vi "example_dynamically_invoking - slave.vi"() -> ()   [LabVIEW 2012]
doc: "This is the Slave VI that is called upon by the controlling Master (example_dynamically_invoking - master.vi). This VI is responsible for handling the communications with the attached hardware while the controlling Master simply issues the appropriate action calls to this one.\n\nProduced By:\n\nChristopher Lemieux\nKod Integrations, LLC\n4835 Marianne Drive\nMount Airy, MD 21771\nhttp://www.kodintegrations.com\nemail: clemieux@kodintegrations.com\nphone: (240) 687-1288"
uses:
  controls/example_dynamically_invoking - slave_actions.ctl
  main_functions/commands.ctl
panel:
  in  "slave_action":T1=enum."initialize"
  out "error out":errorcluster
  in  "error in (no error)":errorcluster
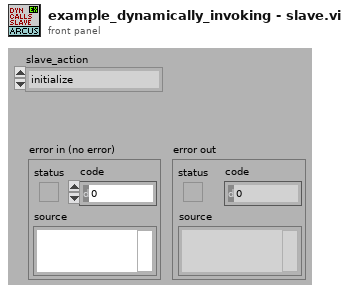
[diagram p1: front panel]
types:
  T1 = typedef "example_dynamically_invoking - slave_actions.ctl" = enum16{"exit", "initialize", "jogConstNeg", "jogConstPos", "stopSlowly"}
  T2 = typedef "commands.ctl" = enum16{"clearErr", "constJogNeg", "constJogPos", "getAccel", "getActualAmp", "getDeviceId", "getDigInputStatus", "getDigInputsStatus", "getDigOutputStatus", "getDigOutputsStatus", "getFirmwareVer", "getHighSpeed", "getIdleAmp", "getLowSpeed", "getMicroStep", "getMotorStatus", "getMoveMode", "getPolarity", "getPosition", "getProdId", "getPwrStatus", "getRunAmp", "getStatus", "homeNeg", "homePos", "moveToPosition", "powerDown", "powerUp", "setAccel", "setDeviceId", "setDigOutput", "setDigOutputs", "setHighSpeed", "setIdleAmp", "setLowSpeed", "setMoveModeAbs", "setMoveModeIncr", "setPolarity", "setPosition", "setRunAmp", "stopNow", "stopSlow", "storeToMem"}
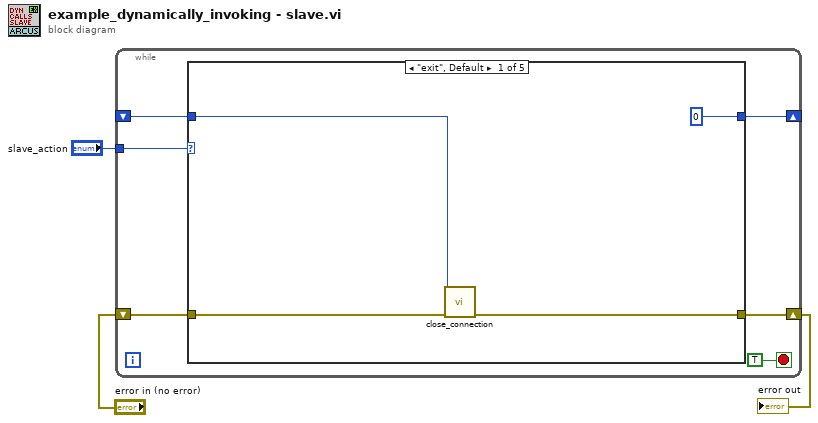
[diagram p0: block diagram]
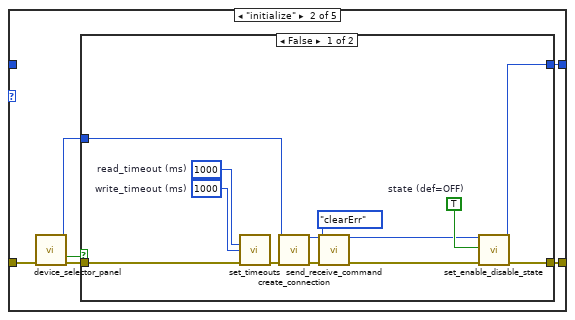
[diagram p2: hidden frame]
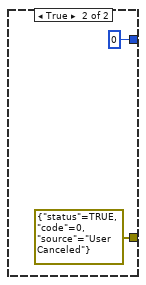
[diagram p3: hidden frame]
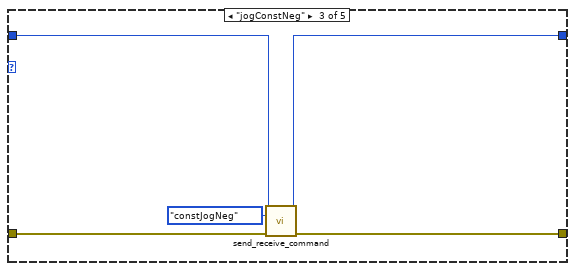
[diagram p4: hidden frame]
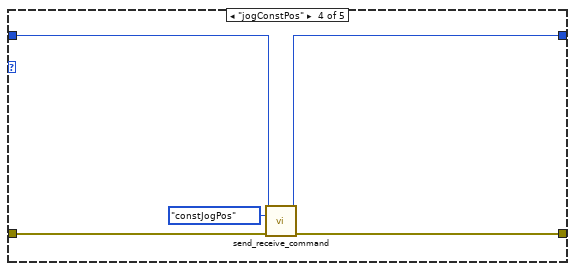
[diagram p5: hidden frame]
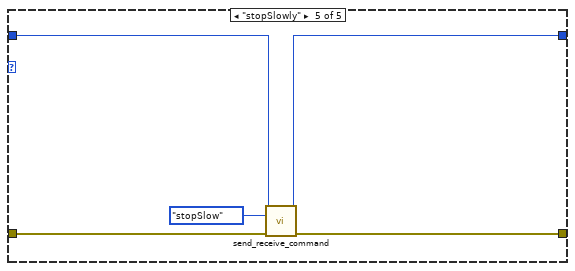
[diagram p6: hidden frame]
diagram:
  n1 = while {
    shift-right: [w7] -> w1
    shift-left: "error in (no error)" -> [w9]
    tunnel: "slave_action" -> [w8]
    shift-right: [w6] -> _
    shift-left: _ -> [w4]
    stop <- TRUE stop-if-true
    n2 = case shown="\"exit\", Default" w8 {
      tunnel: w9 -> [w13 w19 w38 w43 w48]
      tunnel: [w12 w15 w37 w42 w47] -> w7
      tunnel: [0 ("reference (dup)") w14 w35 w40 w45] -> w6
      tunnel: w4 -> [w11 _ w36 w41 w46]
      frame "exit", Default {
        n3 = call "close_connection.vi"("reference"=w11, "error in (no error)"=w13) -> ("error out"=w12:errorcluster)  [unwired: 13 in]
      }
      frame "initialize" {
        n4 = call "device_selector_panel.vi"("error in (no error)"=w19) -> ("index"=w16:i32, "cancel?"=w18:bool, "error out"=w17:errorcluster)  [unwired: 10 in, 2 out]
        n5 = case shown="False" w18 {
          tunnel: w17 -> [w28 _]
          tunnel: w16 -> [w27 _]
          tunnel: [w22 errorcluster {"status"=TRUE, "code"=0, "source"="User Canceled"} ("error out")] -> w15
          tunnel: [w20 0 ("reference (dup)")] -> w14
          frame False {
            w29 = TRUE  # state (def=OFF)
            w31 = 1000  # write_timeout (ms)
            w32 = 1000  # read_timeout (ms)
            n6 = call "set_timeouts.vi"("read_timeout (ms); def=1000"=w32, "write_timeout (ms); def=1000"=w31, "error in (no error)"=w28) -> ("error out"=w26:errorcluster)  [unwired: 12 in]
            n7 = call "create_connection.vi"("device_index (def=0)"=w27, "error in (no error)"=w26) -> ("reference"=w25:i32, "error out"=w24:errorcluster)  [unwired: 12 in]
            n8 = call "send_receive_command.vi"("reference (in)"=w25, "command"=commands."clearErr" ("commands"), "error in (no error)"=w24) -> ("reference (dup)"=w21:i32, "error out"=w23:errorcluster)  [unwired: 8 in, 3 out]
            n9 = call "set_enable_disable_state.vi"("reference (in)"=w21, "state (def=OFF)"=w29, "error in (no error)"=w23) -> ("reference (dup)"=w20:i32, "error out"=w22:errorcluster)  [unwired: 14 in, 1 out]
          }
          frame True {
          }
        }
      }
      frame "jogConstNeg" {
        n10 = call "send_receive_command.vi"("reference (in)"=w36, "command"=commands."constJogNeg" ("commands"), "error in (no error)"=w38) -> ("reference (dup)"=w35:i32, "error out"=w37:errorcluster)  [unwired: 8 in, 3 out]
      }
      frame "jogConstPos" {
        n11 = call "send_receive_command.vi"("reference (in)"=w41, "command"=commands."constJogPos" ("commands"), "error in (no error)"=w43) -> ("reference (dup)"=w40:i32, "error out"=w42:errorcluster)  [unwired: 8 in, 3 out]
      }
      frame "stopSlowly" {
        n12 = call "send_receive_command.vi"("reference (in)"=w46, "command"=commands."stopSlow" ("commands"), "error in (no error)"=w48) -> ("reference (dup)"=w45:i32, "error out"=w47:errorcluster)  [unwired: 8 in, 3 out]
      }
    }
  }
  "error out" <- w1
